vi "Sector Analysis ModuleV2.vi"(11 "Canceled?":bool) -> (0 "New Data? Out":bool, 1 "Analysis Ticks":u32, 2 "State":T1, 4 "Left Sector Edge":u8, 5 "Right Sector Edge":u8)   [LabVIEW 2013]
uses:
  FPGA/Sector/Analysis/Sector Analysis Module Enum.ctl
  <vilib>/rvi/FIFO/Fifo_Resource/nirvififoEmulationReadFpgaImpl.vi
  <vilib>/rvi/DataTransferAndStorage/Container/Common/niFpgaContainerGetUniqueNameForEmu.vi
  FPGA/Globals/Accumulated Sector Intensity.vi
  FPGA/Globals/Sector Parameter Global.vi
  <vilib>/rvi/Emulation/niFpgaSctlEmulationGetInTimedLoop.vi
  <vilib>/rvi/Emulation/niFpgaProcessEmulError.vi
  <vilib>/rvi/FIFO/Fifo_Resource/nirvififoEmulationClearFpgaImpl.vi
  <vilib>/rvi/DataTransferAndStorage/Container/XNode/niFpgaContainer.xnode
  <vilib>/rvi/FIFO/Fifo_Resource/nirvififoEmulationRead.vi
  <vilib>/rvi/FIFO/Fifo_Resource/nirvififoEmulationClear.vi
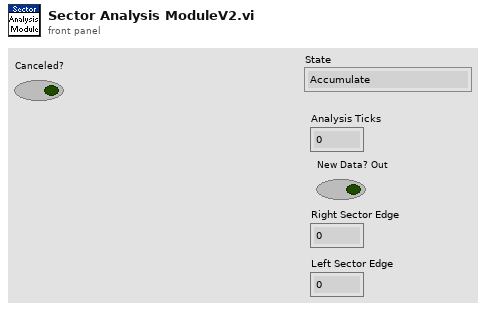
[diagram p1: front panel]
types:
  T1 = typedef "Sector Analysis Module Enum.ctl" = enum16{"Accumulate", "Analysis", "Reset"}
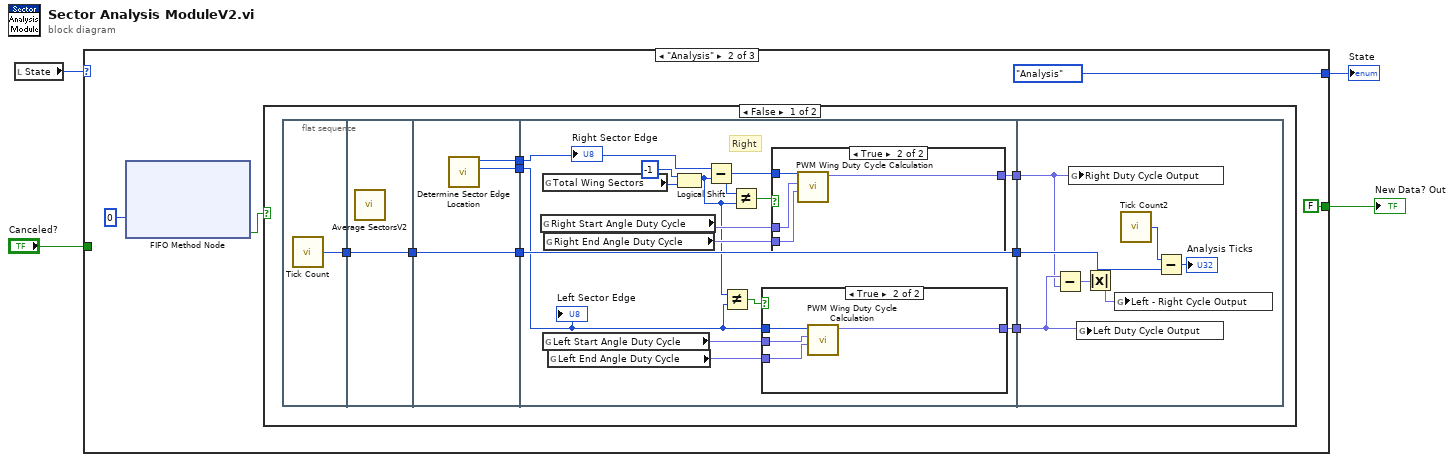
[diagram p0: block diagram]
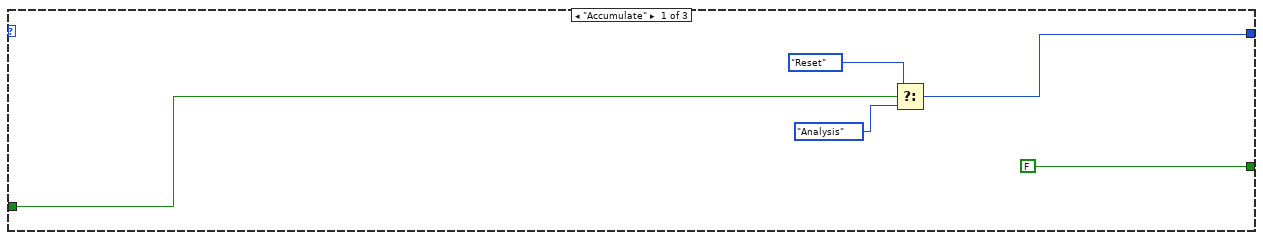
[diagram p2: hidden frame]
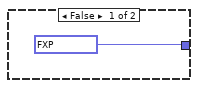
[diagram p3: hidden frame]
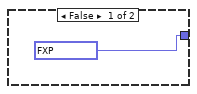
[diagram p4: hidden frame]
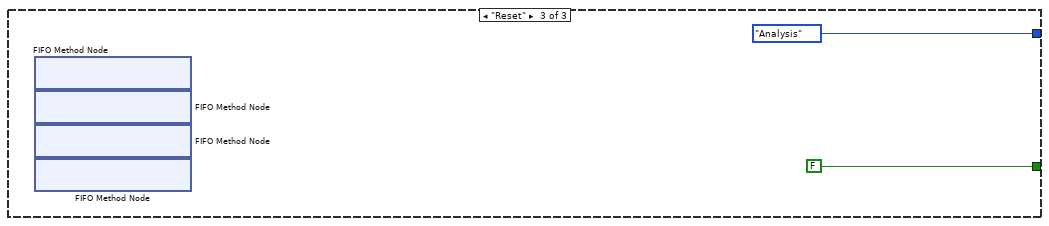
[diagram p6: hidden frame]
diagram:
  n1 = local read "State"() -> (w4:T1)
  n2 = case shown="\"Analysis\"" w4 {
    tunnel: [w8 Sector_Analysis_Module_Enum."Analysis" ("State") Sector_Analysis_Module_Enum."Analysis" ("State")] -> w3
    tunnel: "Canceled?" -> [w9 _ _]
    tunnel: [FALSE ("New Data? Out") FALSE ("New Data? Out") FALSE ("New Data? Out")] -> w1
    frame "Accumulate" {
      n3 = Select(t=Sector_Analysis_Module_Enum."Reset", s=w9, f=Sector_Analysis_Module_Enum."Analysis" ("State")) -> (s? t:f=w8:T1)
    }
    frame "Analysis" {
      n4 = xnode ("FIFO Method Node")("Timeout"=0) -> ("Timed Out?"=w11:bool)  [unwired: 1 in, 2 out]
      n5 = case shown="False" w11 {
        frame False {
          n6 = flat-sequence {
            tunnel: [w22] -> w21
            tunnel: [w23] -> w20
            tunnel: w21 -> [w23]
            tunnel: [w26] -> w19
            tunnel: [w25] -> w18
            tunnel: [w24] -> w17
            tunnel: w20 -> [w24]
            tunnel: [w41] -> w16
            tunnel: w17 -> [w41]
            tunnel: w18 -> [w33]
            tunnel: w19 -> [w38]
            tunnel: [w28] -> w15
            tunnel: [w27] -> w14
            tunnel: w16 -> [w57]
            tunnel: w15 -> [w55]
            tunnel: w14 -> [w54]
            frame #0 {
              n7 = call "Tick Count"() -> ("Tick Count(Ticks)"=w22:u32)
            }
            frame #1 {
              n8 = call "Average SectorsV2.vi"() -> ()  [unwired: 12 in]
            }
            frame #2 {
              n9 = call "Determine Sector Edge Location.vi"() -> ("Left Sector Edge"=w25:u8, "Right Sector Edge"=w26:u8)  [unwired: 10 in]
            }
            frame #3 {
              # "Right"
              n10 = global read "Sector Parameter Global.vi" "Right Start Angle Duty Cycle"() -> (w35:fxp<+,8,0>)
              n11 = global read "Accumulated Sector Intensity.vi" "Total Wing Sectors"() -> (w40:u8)
              n12 = global read "Sector Parameter Global.vi" "Left Start Angle Duty Cycle"() -> (w30:fxp<+,8,0>)
              n13 = global read "Sector Parameter Global.vi" "Right End Angle Duty Cycle"() -> (w34:fxp<+,8,0>)
              n14 = global read "Sector Parameter Global.vi" "Left End Angle Duty Cycle"() -> (w29:fxp<+,8,0>)
              n15 = Logical Shift(y=i16 -1, x=w40) -> (x << y=w32:u8)
              n16 = Subtract(x=w38, y=w32) -> (x-y=w36:u8)
              n17 = Not Equal?(x=w32, y=w33) -> (x != y?=w31:bool)
              n18 = Not Equal?(x=w36, y=w32) -> (x != y?=w37:bool)
              n19 = case shown="True" w31 {
                tunnel: w33 -> [_ w46]
                tunnel: w30 -> [_ w45]
                tunnel: w29 -> [_ w44]
                tunnel: [fxp<+,8,0> 0.99609375 ("Duty Cycle Out") w43] -> w28
                frame False {
                }
                frame True {
                  n20 = call "PWM Wing Duty Cycle Calculation.vi"("End Angle Duty Cycle"=w44, "Start Angle Duty Cycle"=w45, "Sector"=w46) -> ("Duty Cycle Out"=w43:fxp<+,8,0>)  [unwired: 8 in]
                }
              }
              n21 = case shown="True" w37 {
                tunnel: w36 -> [_ w51]
                tunnel: w35 -> [_ w50]
                tunnel: w34 -> [_ w49]
                tunnel: [fxp<+,8,0> 0.99609375 ("Duty Cycle Out") w48] -> w27
                frame False {
                }
                frame True {
                  n22 = call "PWM Wing Duty Cycle Calculation.vi"("End Angle Duty Cycle"=w49, "Start Angle Duty Cycle"=w50, "Sector"=w51) -> ("Duty Cycle Out"=w48:fxp<+,8,0>)  [unwired: 8 in]
                }
              }
              "Right Sector Edge" <- w38
              "Left Sector Edge" <- w33
            }
            frame #4 {
              n23 = Subtract(x=w55, y=w54) -> (x-y=w53:fxp<+/-,9,1>)
              n24 = global write "Sector Parameter Global.vi" "Right Duty Cycle Output"(w54) -> ()
              n25 = global write "Sector Parameter Global.vi" "Left Duty Cycle Output"(w55) -> ()
              n26 = Absolute Value(x=w53) -> (abs(x)=w52:fxp<+,8,0>)
              n27 = global write "Sector Parameter Global.vi" "Left - Right Cycle Output"(w52) -> ()
              n28 = call "Tick Count2"() -> ("Tick Count(Ticks)"=w58:u32)
              n29 = Subtract(x=w58, y=w57) -> (x-y=→"Analysis Ticks":u32)
            }
          }
        }
        frame True {
        }
      }
    }
    frame "Reset" {
      n30 = xnode ("FIFO Method Node")() -> ()  [unwired: 1 in, 1 out]
      n31 = xnode ("FIFO Method Node")() -> ()  [unwired: 1 in, 1 out]
      n32 = xnode ("FIFO Method Node")() -> ()  [unwired: 1 in, 1 out]
      n33 = xnode ("FIFO Method Node")() -> ()  [unwired: 1 in, 1 out]
    }
  }
  "State" <- w3
  "New Data? Out" <- w1
